vi "Write Header - SET parameters.vi"(8 "error in (no error)":errorcluster, 11 "Save Image in":refnum<class "Save Image.lvclass">) -> (0 "error out":errorcluster, 3 "Save Image out":refnum<class "Save Image.lvclass">)   [LabVIEW 2018, in "Save Image.lvclass"]
uses:
  Save Image.lvclass
  Save Image.lvclass/Save Image.ctl
  Interface/Interface.lvclass/Interface.ctl
  Simulated_Header/write keyword - integer.vi
  Simulated_Header/write keyword - string.vi
  Simulated_Header/write keyword - float.vi
  Simulated_Header/write keyword - boolean.vi
  Interface/Interface.lvclass
  <vilib>/Utility/Data Type/NI_Data Type.lvlib
  Simulated_Header/Simulated_Header.lvclass
panel:
  out "Previous SET parameters":T1
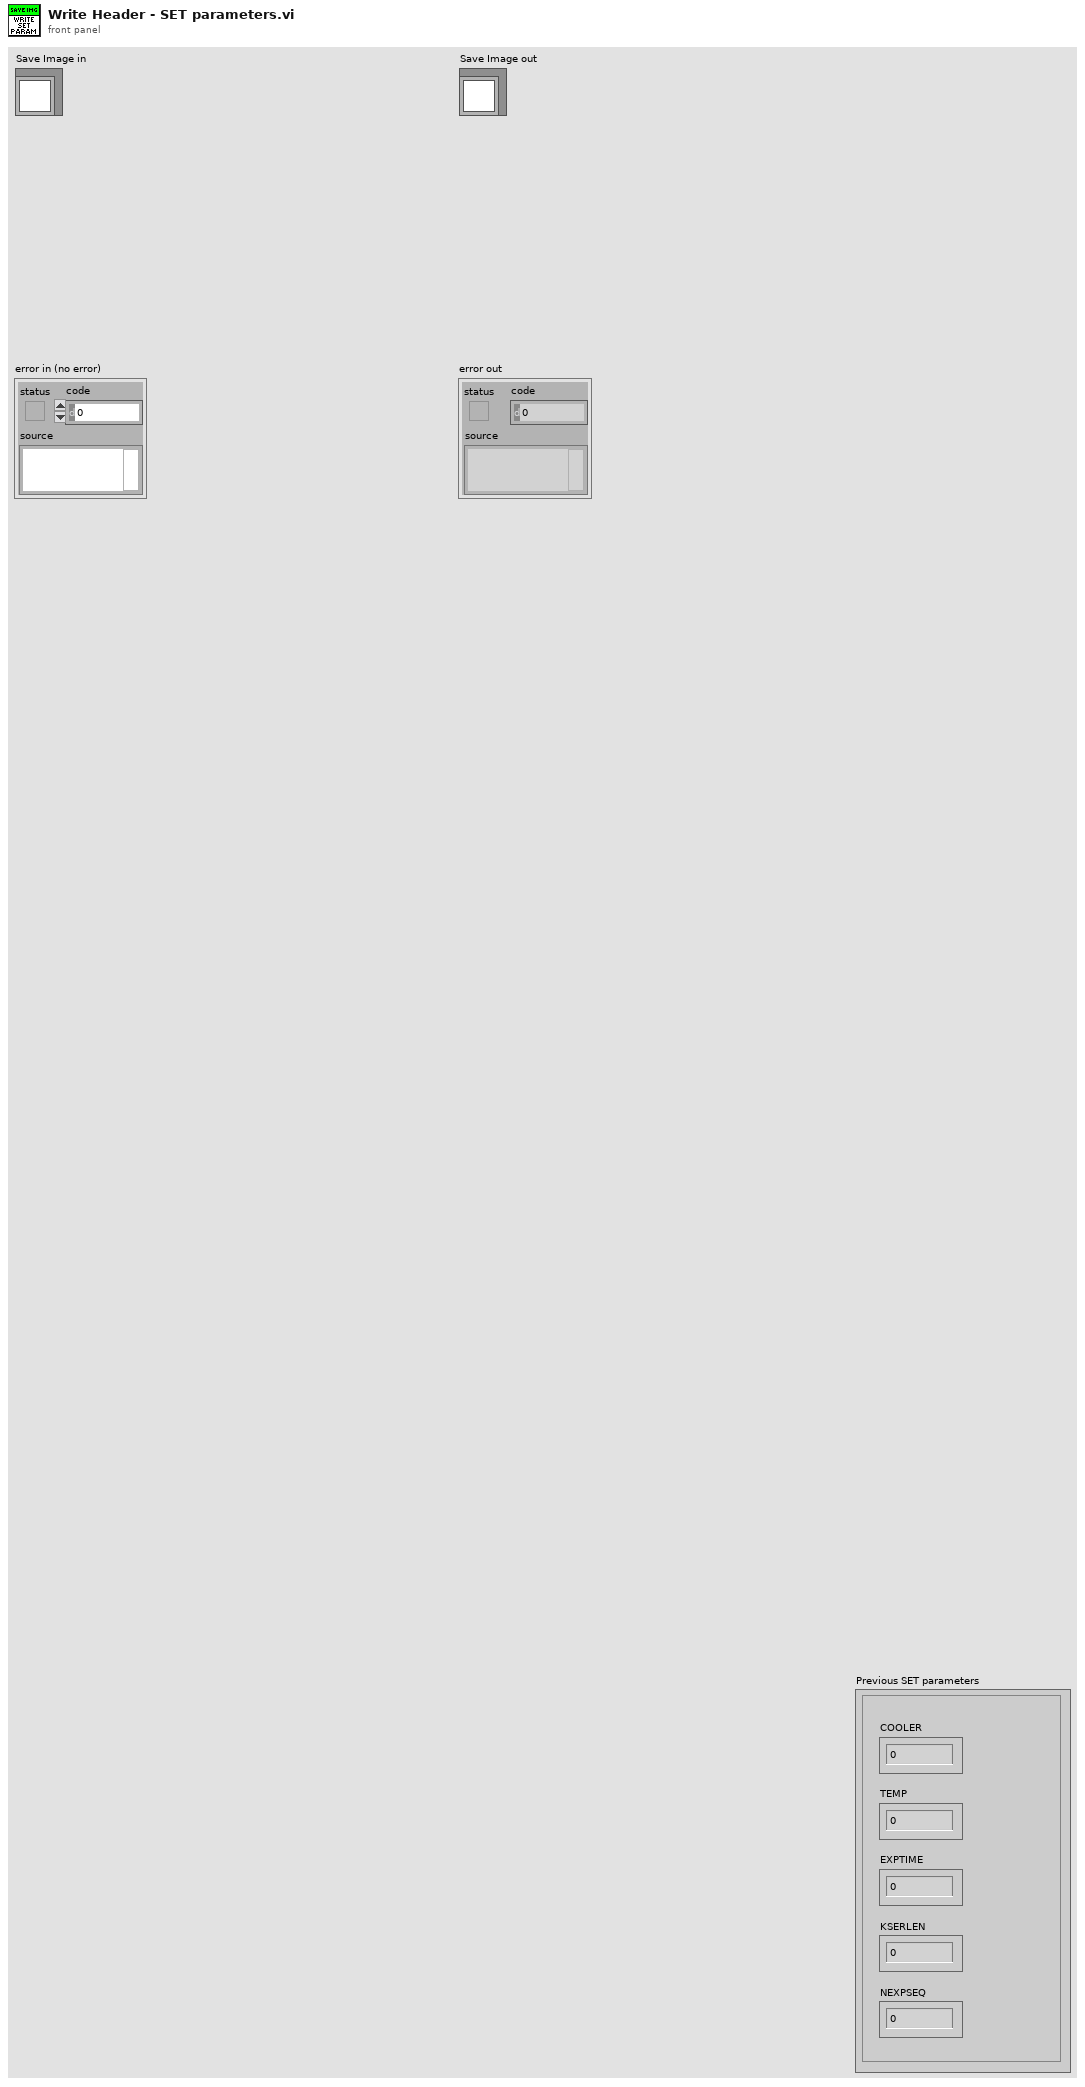
[diagram p1: front panel]
types:
  T1 = cluster{"COOLER":u16, "TEMP":i32, "EXPTIME":dbl, "KSERLEN":u32, "NEXPSEQ":u32}
  T2 = cluster{"COOLER_POWER_STATUS":u16, "TEMP":i32, "EXPTIME":sgl, "#FRAMES":u32, "#CUBES":u32}
  T3 = typedef "NI_Data Type.lvlib/Data Type.ctl" = enum8{"Invalid Type", "Void", "I8", "I16", "I32", "I64", "U8", "U16", "U32", "U64", "Single Float", "Double Float", "Extended Float", "Single Complex", "Double Complex", "Extended Complex", "Enum U8", "Enum U16", "Enum U32", "Enum U64", "Single Float With Unit", "Double Float With Unit", "Extended Float With Unit", "Single Complex with Unit", "Double Complex with Unit", "Extended Complex with Unit", "Boolean", "String", "Path", "Picture", "Tag", "Array", "Cluster", "Variant", "LV Variant", "Waveform", "Timestamp", "Digital Waveform", "Digital Data", "ExpressData", "Refnum", "External Data", "VI", "Poly VI", "LabVIEW Class Instance", "Fixed Point"}
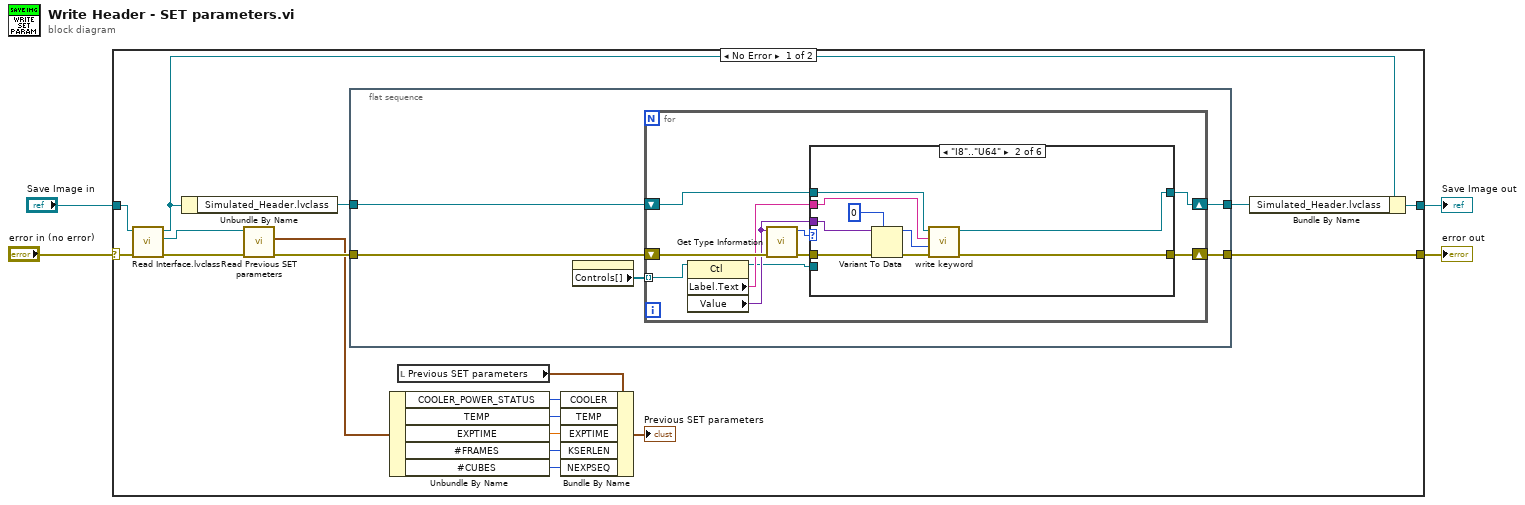
[diagram p0: block diagram]
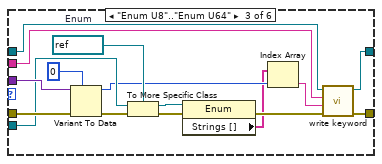
[diagram p3: hidden frame]
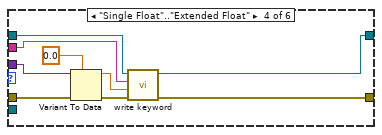
[diagram p4: hidden frame]
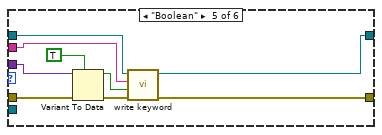
[diagram p5: hidden frame]
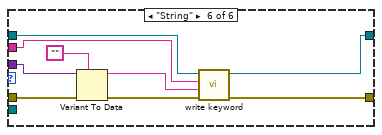
[diagram p6: hidden frame]
diagram:
  n1 = case shown="No Error" "error in (no error)" {
    selector: "error in (no error)" -> [w22 w92]
    tunnel: [w14 w92] -> w3
    tunnel: [w15 w93] -> w1
    tunnel: "Save Image in" -> [w21 w93]
    frame No Error {
      n2 = call "Read Interface.lvclass.vi"("error in (no error)"=w22, "Save Image in"=w21) -> ("error out"=w19:errorcluster, "Interface.lvclass"=w20:refnum<class "Interface.lvclass">, "Save Image out"=w18:refnum<class "Save Image.lvclass">)  [unwired: 7 in]
      n3 = Unbundle By Name(w18) -> ("Simulated_Header.lvclass"=w17:refnum<class "Simulated_Header.lvclass">)
      n4 = call "Read Previous SET parameters.vi"("error in (no error)"=w19, "Interface in"=w20) -> ("error out"=w16:errorcluster, "Previous SET parameters"=w13:T2)  [unwired: 7 in, 1 out]
      n5 = flat-sequence {
        tunnel: [w27] -> w14
        tunnel: w17 -> [w26]
        tunnel: [w25] -> w5
        tunnel: w16 -> [w24]
        frame #0 {
          n6 = property on="Previous SET parameters" class="Clust (strict)"() -> ("Controls[]"=w23:refnum<vi>[])  [unwired: 2 in, 2 out]
          n7 = for {
            shift-right: [w33] -> w25
            shift-left: w26 -> [w31]
            shift-right: [w34] -> w27
            shift-left: w24 -> [w37]
            tunnel: w23 -> [w30] mode=indexing
            n8 = property class="Ctl"(reference=w30) -> (reference out=w29:refnum<vi>, "Label.Text"=w35:string, "Value"=w32:variant)  [unwired: 1 in, 1 out]
            n9 = call <vilib>:"Get Type Information.vi"("error in (no error)"=w37, "Variant"=w32) -> ("error out"=w36:errorcluster, "Type"=w28:T3)  [unwired: 5 in, 3 out]
            n10 = case shown="\"I8\"..\"U64\"" w28 {
              tunnel: w36 -> [w39 w48 w64 w73 w82 w91]
              tunnel: w35 -> [_ w44 w62 w69 w78 w87]
              tunnel: [w39 w43 w61 w68 w77 w86] -> w34
              tunnel: [w38 w42 w60 w67 w76 w85] -> w33
              tunnel: w32 -> [_ w41 w59 w66 w75 w84]
              tunnel: w31 -> [w38 w40 w58 w65 w74 w83]
              tunnel: w29 -> [_ _ w56 _ _ _]
              frame "Invalid Type", Default {
              }
              frame "I8".."U64" {
                n11 = Variant To Data(error in=w48, type=0, Variant=w41) -> (data=w45:i32, error out=w46:errorcluster)
                n12 = call-poly "write keyword.vi"("error in (no error)"=w46, "Value"=w45, "keyword"=w44, "Simulated_Header in"=w40) -> ("error out"=w43:errorcluster, "Simulated_Header out"=w42:refnum<class "Simulated_Header.lvclass">)  [unwired: 6 in]
              }
              frame "Enum U8".."Enum U64" {
                w52 = refnum<vi> refnum  # Enum
                n13 = Variant To Data(error in=w64, type=0, Variant=w59) -> (data=w51:i32, error out=w55:errorcluster)
                n14 = To More Specific Class(target class=w52, reference=w56, error in=w55) -> (specific class reference=w54:refnum<vi>, error out=w53:errorcluster)
                n15 = property on="Property Node" class="Enum"(reference=w54, error in=w53) -> (error out=w57:errorcluster, "Strings []"=w50:string[])  [unwired: 1 out]
                n16 = Index Array(array=w50, index=w51) -> (element=w49:string)
                n17 = call-poly "write keyword.vi"("error in (no error)"=w57, "value"=w49, "keyword"=w62, "Simulated_Header in"=w58) -> ("error out"=w61:errorcluster, "Simulated_Header out"=w60:refnum<class "Simulated_Header.lvclass">)  [unwired: 6 in]
              }
              frame "Single Float".."Extended Float" {
                n18 = Variant To Data(error in=w73, type=0.0, Variant=w66) -> (data=w70:dbl, error out=w71:errorcluster)
                n19 = call-poly "write keyword.vi"("error in (no error)"=w71, "Value"=w70, "keyword"=w69, "Simulated_Header in"=w65) -> ("error out"=w68:errorcluster, "Simulated_Header out"=w67:refnum<class "Simulated_Header.lvclass">)  [unwired: 6 in]
              }
              frame "Boolean" {
                n20 = Variant To Data(error in=w82, type=TRUE, Variant=w75) -> (data=w79:bool, error out=w80:errorcluster)
                n21 = call-poly "write keyword.vi"("error in (no error)"=w80, "value"=w79, "keyword"=w78, "Simulated_Header in"=w74) -> ("error out"=w77:errorcluster, "Simulated_Header out"=w76:refnum<class "Simulated_Header.lvclass">)  [unwired: 6 in]
              }
              frame "String" {
                n22 = Variant To Data(error in=w91, type="", Variant=w84) -> (data=w88:string, error out=w89:errorcluster)
                n23 = call-poly "write keyword.vi"("error in (no error)"=w89, "value"=w88, "keyword"=w87, "Simulated_Header in"=w83) -> ("error out"=w86:errorcluster, "Simulated_Header out"=w85:refnum<class "Simulated_Header.lvclass">)  [unwired: 6 in]
              }
            }
          }
        }
      }
      n24 = Unbundle By Name(w13) -> ("COOLER_POWER_STATUS"=w10:u16, "TEMP"=w9:i32, "EXPTIME"=w8:sgl, "#FRAMES"=w7:u32, "#CUBES"=w6:u32)
      n25 = local read "Previous SET parameters"() -> (w11:T1)
      n26 = Bundle By Name(cluster=w11, "COOLER"=w10, "TEMP"=w9, "EXPTIME"=w8, "KSERLEN"=w7, "NEXPSEQ"=w6) -> (→"Previous SET parameters":T1)
      n27 = Bundle By Name(cluster=w18, "Simulated_Header.lvclass"=w5) -> (w15:refnum<class "Save Image.lvclass">)
    }
    frame Error {
    }
  }
  "error out" <- w3
  "Save Image out" <- w1
